vi "Send Message to Notebook.vi"(5 "Text Formatting":T1={"Font"="Default", "Text Color"=enum."Unchanged", "Text Background Color"=enum."Unchanged", "Text Style"=enum."Regular", "Font Size (Points)"=-1.0, "Text Alignment"=0} {"Text Alignment" items=["Left", "Right", "Center"]}, 6 "Error In":errorcluster, 7 "Message":string, 9 "Notebook Queue":refnum<queue>) -> (0 "Error Out":errorcluster, 3 "Notebook Queue":refnum<queue>)   [LabVIEW 2021, in "Notebook.lvlib"]
doc: "This VI executes no matter what the <B>Error in</B> value is.\nThe error is passed unchanged to <B>Error out</B>, or, if there is an error when sending the message, with that new error appended to the incoming one."
uses:
  Notebook.lvlib
  Notebook Action Q Element.ctl
  Notebook Action List.ctl
  Rich Text Box/Text Formatting.ctl
  Rich Text Box/Text Colors.ctl
  Rich Text Box/Formatted Text.ctl
  Rich Text Box/Rich Text Box.lvlib
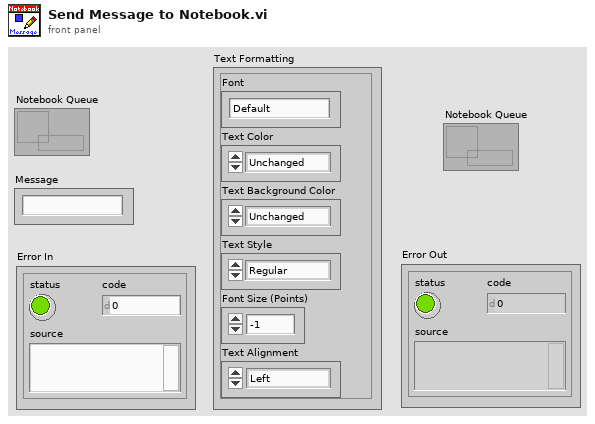
[diagram p1: front panel]
types:
  T1 = typedef "Rich Text Box.lvlib/Text Formatting.ctl" = cluster{"Font":string, "Text Color":T2, "Text Background Color":T2, "Text Style":enum16{"Regular", "Bold", "Italic", "Underline", "Strikeout"}, "Font Size (Points)":dbl, "Text Alignment":i32}
  T2 = typedef "Rich Text Box.lvlib/Text Colors.ctl" = enum16{"Unchanged", "Black", "Blue", "Brown", "Gray", "Green", "Orange", "Pink", "Red", "White"}
  T3 = typedef "Rich Text Box.lvlib/Formatted Text.ctl" = cluster{"Text":string, "Text Formatting":T1}
  T4 = typedef "Notebook.lvlib/Notebook Action Q Element.ctl" = cluster{"Action":T5, "Variant":variant}
  T5 = typedef "Notebook.lvlib/Notebook Action List.ctl" = enum16{"Idle", "Init", "Check Content Change", "User added content", "Program added text", "Program added Picture ", "Save Notebook", "Quit", "Open", "Close", "Update Window Title"}
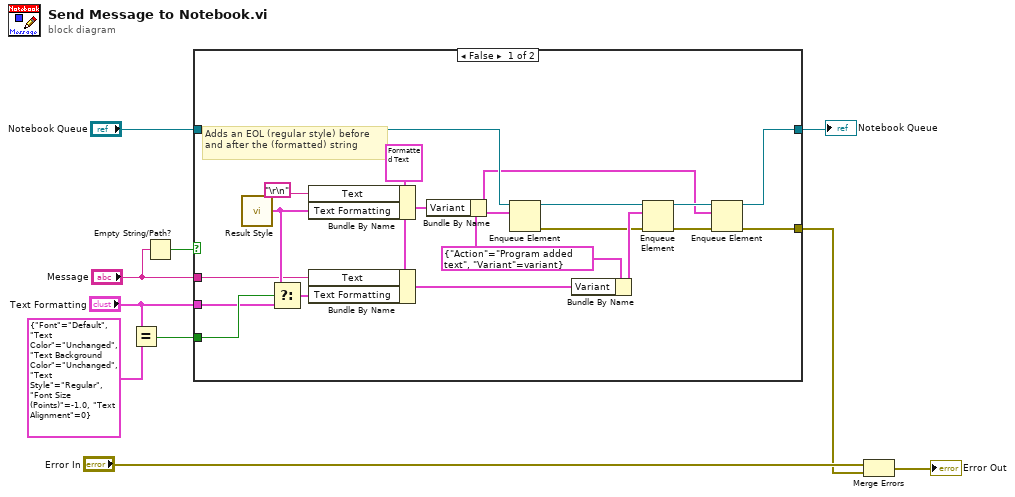
[diagram p0: block diagram]
diagram:
  n1 = Equal?(x="Text Formatting", y=T1 {"Font"="Default", "Text Color"=enum."Unchanged", "Text Background Color"=enum."Unchanged", "Text Style"=enum."Regular", "Font Size (Points)"=-1.0, "Text Alignment"=0} ("Text Formatting")) -> (x = y?=w9:bool)
  n2 = Empty String/Path?(string/path="Message") -> (empty?=w5:bool)
  n3 = case shown="False" w5 {
    tunnel: "Notebook Queue" -> [w28 w30]
    tunnel: w9 -> [w17 _]
    tunnel: "Text Formatting" -> [w14 _]
    tunnel: "Message" -> [w13 _]
    tunnel: [w12 _] -> w2
    tunnel: [w11 w30] -> w1
    frame False {
      w22 = T3 {"Text"="", "Text Formatting"={"Font"="Default", "Text Color"=enum."Unchanged", "Text Background Color"=enum."Unchanged", "Text Style"=enum."Regular", "Font Size (Points)"=-1.0, "Text Alignment"=0}} ("Formatted Text")
      w26 = T4 {"Action"=enum."Program added text", "Variant"=variant} ("element")
      # "Adds an EOL (regular style) before and after the (formatted) string"
      n4 = call "Result Style.vi"() -> ("Default Text Formatting"=w16:T1)
      n5 = Select(t=w16, s=w17, f=w14) -> (s? t:f=w15:T1)
      n6 = Bundle By Name(cluster=w22, "Text"="\r\n", "Text Formatting"=w16) -> (w24:T3)
      n7 = Bundle By Name(cluster=w22, "Text"=w13, "Text Formatting"=w15) -> (w18:T3)
      n8 = Bundle By Name(cluster=w26, "Variant"=w24) -> (w19:T4)
      n9 = Enqueue Element(queue=w28, element=w19) -> (queue out=w27:refnum<queue>, error out=w23:errorcluster)  [unwired: 2 in, 1 out]
      n10 = Bundle By Name(cluster=w26, "Variant"=w18) -> (w29:T4)
      n11 = Enqueue Element(queue=w27, element=w29, error in (no error)=w23) -> (queue out=w20:refnum<queue>, error out=w21:errorcluster)  [unwired: 1 in, 1 out]
      n12 = Enqueue Element(queue=w20, element=w19, error in (no error)=w21) -> (queue out=w11:refnum<queue>, error out=w12:errorcluster)  [unwired: 1 in, 1 out]
    }
    frame True {
    }
  }
  "Notebook Queue" <- w1
  n13 = Merge Errors("Error In", w2) -> (→"Error Out":errorcluster)
